vi "getMirrorPosition.vi"(6 "Delay between send and receive [ms]":i32=100, 8 "error in (no error)":errorcluster, 10 "locationId":T1=enum."1 = Mirror 2 (Exit)", 11 "Monochromator in":refnum<class "Monochromator.lvclass">) -> (0 "error out":errorcluster, 2 "Position":T2, 3 "Monochromator out":refnum<class "Monochromator.lvclass">)   [LabVIEW 2023, in "Monochromator.lvclass"]
uses:
  Monochromator.lvclass
  MirrorPositionEnum.ctl
  MirrorPosition.ctl
  2283113d-39d5-42fa-820e-b0e09e745b74.vi
  d9b87029-586e-44ee-a6e5-d4a5e0edce38.vi
  b59fd1e7-dcda-425c-bd6c-61aafb79e7f4.vi
  <vilib>/JDP Science/JSONtext/Variant to JSON Text.vi
  <vilib>/JDP Science/JSONtext/Set Item.vi
  <vilib>/JDP Science/JSONtext/JSON text to Variant.vi
  <vilib>/JDP Science/JSONtext/LVClass Serializer/JSONtext LVClass Serializer.lvclass
  Monochromator.lvclass/Monochromator.ctl
  GenericDevice/GenericDevice.lvclass
  <vilib>/IlluminatedG/lv-web-crypto/lv-json/JSON/JSON.lvlib
  CCD/MirrorLocationEnum.ctl
panel:
  # "Connector Pane"
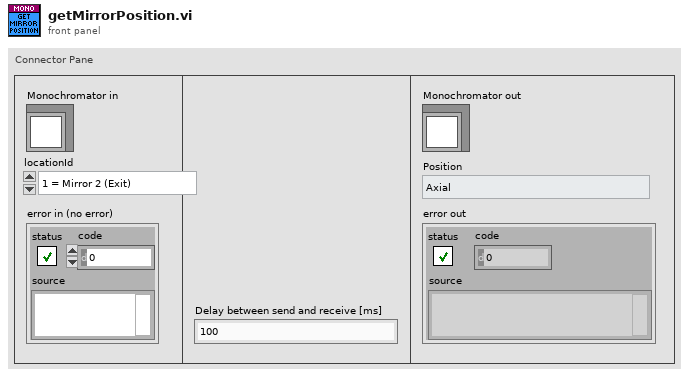
[diagram p1: front panel]
types:
  T1 = typedef "Monochromator.lvclass/MirrorLocationEnum.ctl" = enum32{"0 = Mirror 1 (Entrance) ", "1 = Mirror 2 (Exit)"}
  T2 = typedef "Monochromator.lvclass/MirrorPositionEnum.ctl" = enum16{"Axial", "Lateral", "unknown"}
  T3 = typedef "Monochromator.lvclass/MirrorPosition.ctl" = cluster{"position":i32}
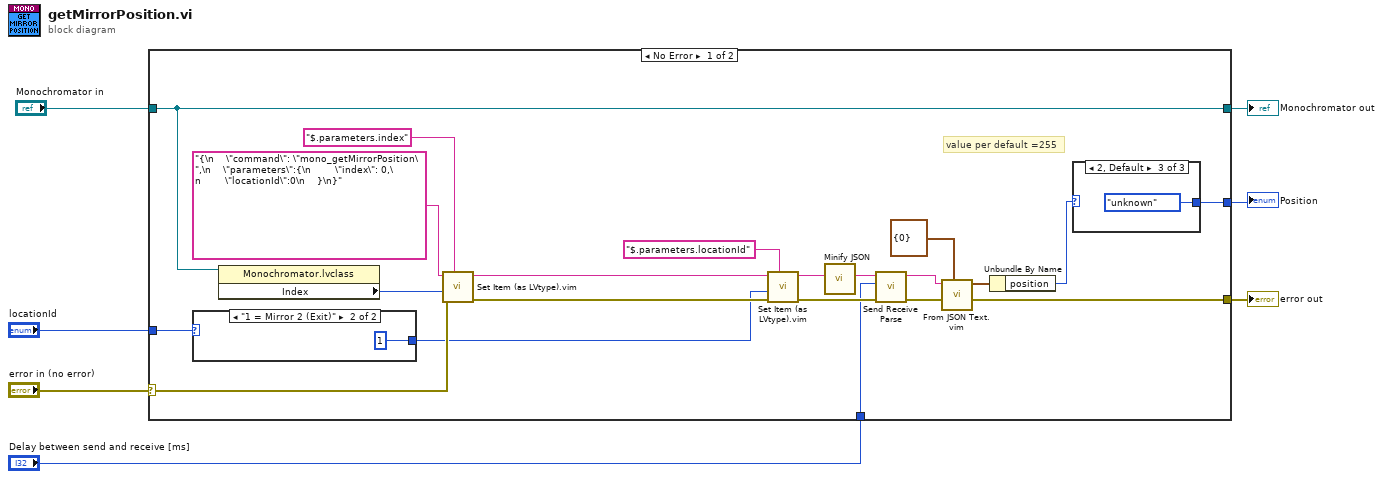
[diagram p0: block diagram]
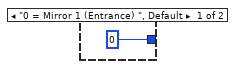
[diagram p2: hidden frame]
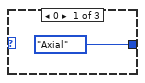
[diagram p3: hidden frame]
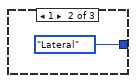
[diagram p4: hidden frame]
diagram:
  n1 = case shown="No Error" "error in (no error)" {
    selector: "error in (no error)" -> [w13 w35]
    tunnel: [w27 w35] -> w6
    tunnel: [w14 w34] -> w4
    tunnel: "Monochromator in" -> [w14 w34]
    tunnel: [w18 _] -> w3
    tunnel: "locationId" -> [w8 _]
    tunnel: "Delay between send and receive [ms]" -> [w10 _]
    frame No Error {
      # "value per default =255"
      n2 = case shown="\"1 = Mirror 2 (Exit)\"" w8 {
        tunnel: [0 1] -> w9
        frame "0 = Mirror 1 (Entrance) ", Default {
        }
        frame "1 = Mirror 2 (Exit)" {
        }
      }
      n3 = property class="Monochromator.lvclass"(reference=w14) -> ("Index"=w17:i32)  [unwired: 1 in, 2 out]
      n4 = call "Set Item (as LVtype).vim"("$Path or Item Name"="$.parameters.index", "error in (no error)"=w13, "Anything"=w17, "JSON"="{\n    \"command\": \"mono_getMirrorPosition\",\n    \"parameters\":{\n        \"index\": 0,\n        \"locationId\":0\n    }\n}") -> ("error out"=w12:errorcluster, "<JSON>"=w11:string)  [unwired: 4 in, 1 out]
      n5 = call "Set Item (as LVtype).vim"("$Path or Item Name"="$.parameters.locationId", "error in (no error)"=w12, "Anything"=w9, "JSON"=w11) -> ("error out"=w26:errorcluster, "<JSON>"=w23:string)  [unwired: 4 in, 1 out]
      n6 = call <vilib>:"Minify JSON.vi"("JSON String"=w23) -> ("Minified JSON"=w22:string)  [unwired: 10 in]
      n7 = call "Send Receive Parse.vi"("error in"=w26, "Delay between send and receive [ms]"=w10, "<JSON>"=w22) -> ("error out"=w24:errorcluster, "results-JSON string"=w25:string)  [unwired: 6 in, 1 out]
      n8 = call "From JSON Text.vim"("Data Type and Default Value"=T3 {"position"=0} ("Mirror Orientation"), "error in (no error)"=w24, "JSON"=w25) -> ("error out"=w27:errorcluster, "Data out"=w21:T3)  [unwired: 7 in]
      n9 = Unbundle By Name(w21) -> ("position"=w19:i32)
      n10 = case shown="2, Default" w19 {
        tunnel: [MirrorPositionEnum."Axial" ("Position") MirrorPositionEnum."Lateral" ("Position") MirrorPositionEnum."unknown" ("Position")] -> w18
        frame 0 {
        }
        frame 1 {
        }
        frame 2, Default {
        }
      }
    }
    frame Error {
    }
  }
  "error out" <- w6
  "Monochromator out" <- w4
  "Position" <- w3
